vi "End Other VI.vi"(8 "error in (no error)":errorcluster, 10 "TCP Connection":refnum<k5>, 11 "queue in":refnum<queue>) -> (0 "error out":errorcluster)   [LabVIEW 2020]
uses:
  Queue Type.ctl
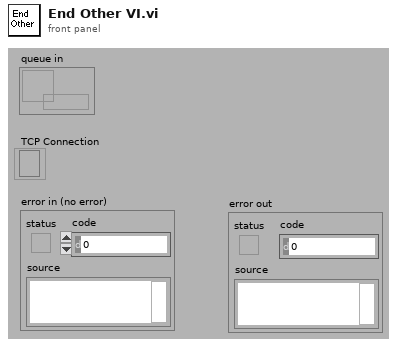
[diagram p1: front panel]
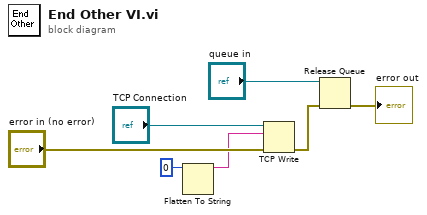
[diagram p0: block diagram]
diagram:
  n1 = Flatten To String(anything=0) -> (data string=w1:string)  [unwired: 1 in, 4 out]
  n2 = TCP Write(connection ID="TCP Connection", data in=w1, error in (no error)="error in (no error)") -> (error out=w3:errorcluster)  [unwired: 3 out]
  n3 = Release Queue(queue="queue in", error in (no error)=w3) -> (error out=→"error out":errorcluster)  [unwired: 3 out]
